vi "Single Engine Main.vi"() -> ()   [LabVIEW 2013]
uses:
  <vilib>/NI/Module Execution Interface/Engine Runtime/Execution States.ctl
  <vilib>/NI/Module Execution Interface/Engine Runtime/Engine Runtime Interface.lvclass
  Framework Configuration Classes/target runtime/PL_Target Runtime.lvclass
  Framework Configuration Classes/platypus configuration/PLConfigurationSerializer.lvlib
  <vilib>/rvi/interface/nirviOpenFPGA/nirviOpenFPGA.xnode
  <vilib>/NI/Tag Bus Module Framework/FPGA manager/FPGA manager.lvlib
  <vilib>/NI/Tag Bus Module Framework/FPGA manager/methods.ctl
  <vilib>/userdefined/High Color/nirio_resource_hc.ctl
panel:
  out "final error":errorcluster
  in  "stop":bool
  out "runtime error":errorcluster
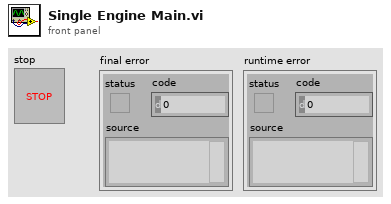
[diagram p1: front panel]
types:
  T1 = typedef "nirio_resource_hc.ctl" = tag
  T2 = typedef "FPGA manager.lvlib/methods.ctl" = enum16{"initialize bitfile", "cache bitfile", "locate bitfile", "close bitfile"}
  T3 = typedef "PLConfigurationSerializer.lvlib/file format.ctl" = cluster{"version":string, "data":string}
  T4 = typedef "PLConfigurationSerializer.lvlib/1_0_0_0 format.ctl" = cluster{"system":T5, "database":T8[]}
  T5 = typedef "PLConfigurationSerializer.lvlib/system hierarchy.ctl" = cluster{"system ID":string, "targets":T6[]}
  T6 = typedef "PLConfigurationSerializer.lvlib/target hierarchy.ctl" = cluster{"target ID":string, "engines":T7[]}
  T7 = typedef "PLConfigurationSerializer.lvlib/engine hierarchy.ctl" = cluster{"engine ID":string, "modules IDs":string[]}
  T8 = typedef "PLConfigurationSerializer.lvlib/configuration database.ctl" = cluster{"ID":string, "display name":string, "class":string, "version":string, "data":string}
  T9 = typedef "PLConfigurationSerializer.lvlib/targets cluster.ctl" = cluster{"Target Configuration":refnum<class "PL_Target Configuration.lvclass">, "engines":T10[]}
  T10 = typedef "PLConfigurationSerializer.lvlib/engines cluster.ctl" = cluster{"engine configuration":refnum<class "engine configuration.lvclass">, "modules":refnum<class "TBM module configuration.lvclass">[]}
  T11 = typedef "Engine Runtime Interface.lvclass/Execution States.ctl" = enum16{"Initializing", "Paused (Initialized)", "Running", "Set Safe Outputs", "Uninitializing", "Stopped (Uninitialized)", "Error (Uninitialized)", "Safe State (Uninitialized)", "Closed"}
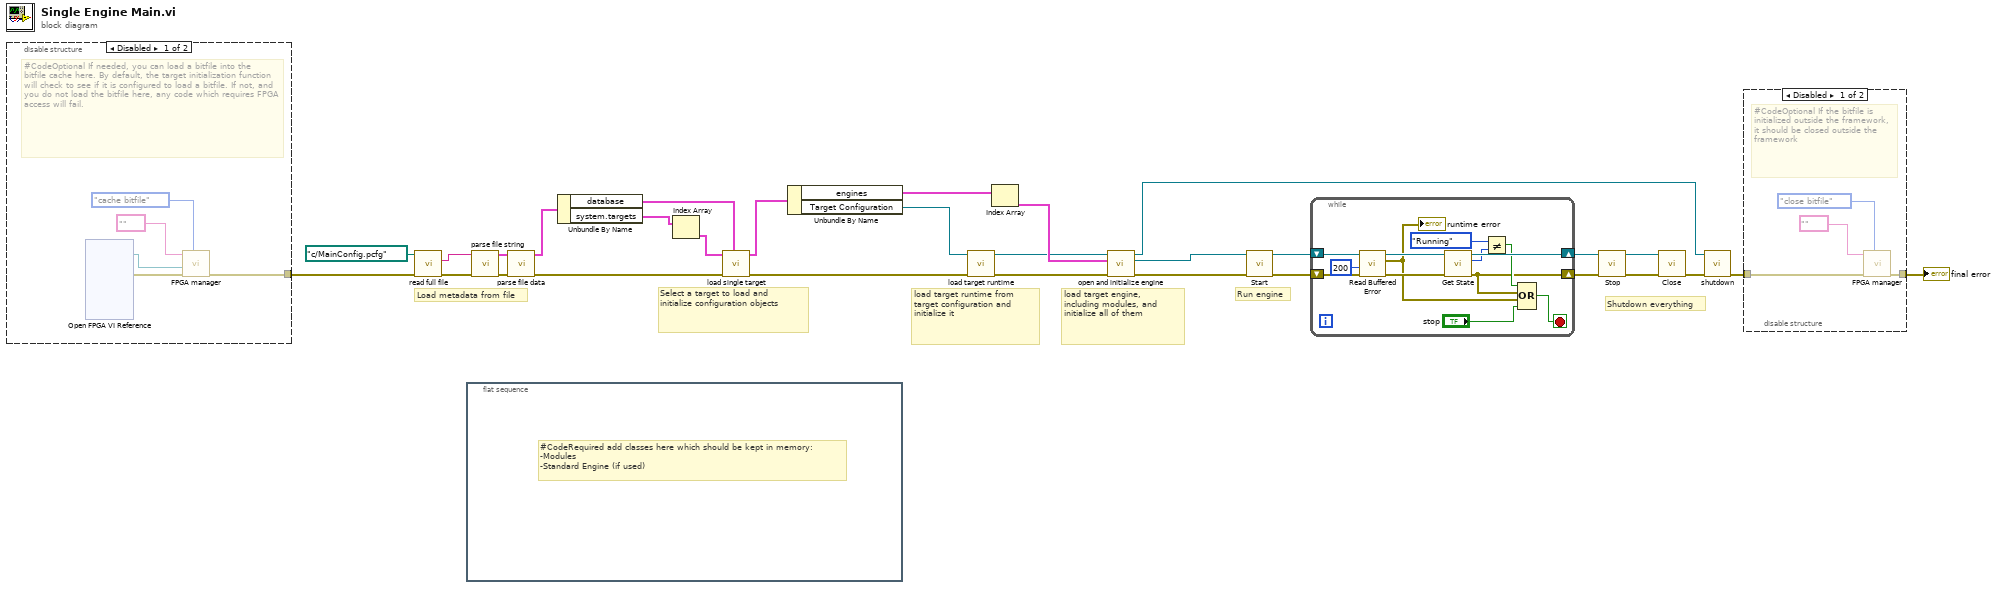
[diagram p0: block diagram]
diagram:
  # "Shutdown everything"
  # "Run engine"
  # "load target engine, including modules, and initialize all of them"
  # "load target runtime from target configuration and initialize it"
  # "Select a target to load and initialize configuration objects"
  # "Load metadata from file"
  n1 = disable-structure shown="Disabled" {
    disable-tunnel: [w31 _] -> w3
    frame Disabled {
      # "#CodeOptional If needed, you can load a bitfile into the bitfile cache here. By default, the target initialization function will check to see if it is configured to load a bitfile. If not, and you do not load the bitfile here, any code which requires FPGA access will fail."
      n2 = xnode "Open FPGA VI Reference"() -> ("FPGA VI Reference Out"=w34:refnum<k20>, "error out"=w35:errorcluster)  [unwired: 2 in]
      n3 = call <vilib>:"FPGA manager.vi"("action"=methods."cache bitfile", "error in"=w35, "bitfile to cache"=w34, "RIO resource"=T1 "") -> ("error out"=w31:errorcluster)  [unwired: 5 in, 2 out]
    }
    frame Enabled {
    }
  }
  n4 = call "read full file.vi"("error in"=w3, "file path"=path "c:/MainConfig.pcfg") -> ("error out"=w20:errorcluster, "data"=w21:string)  [unwired: 8 in]
  n5 = flat-sequence {
    frame #0 {
      # "#CodeRequired add classes here which should be kept in memory:\n-Modules\n-Standard Engine (if used)"
      # "Add classes here to be in memory"
    }
  }
  n6 = call "parse file string.vi"("error in"=w20, "data string"=w21) -> ("error out"=w22:errorcluster, "file format"=w23:T3)  [unwired: 8 in]
  n7 = call "parse file data.vi"("error in"=w22, "file format"=w23) -> ("error out"=w18:errorcluster, "file information"=w19:T4)  [unwired: 8 in]
  n8 = Unbundle By Name(w19) -> ("database"=w17:T8[], "system.targets"=w16:T6[])
  n9 = Index Array(array=w16) -> (element=w15:T6)  [unwired: 1 in]
  n10 = call "load single target.vi"("database in"=w17, "error in"=w18, "target to load"=w15) -> ("error out"=w6:errorcluster, "targets cluster out"=w14:T9)  [unwired: 7 in]
  n11 = Unbundle By Name(w14) -> ("engines"=w13:T10[], "Target Configuration"=w7:refnum<class "PL_Target Configuration.lvclass">)
  n12 = call "load target runtime.vi"("error in"=w6, "target configuration"=w7) -> ("error out"=w5:errorcluster, "target runtime"=w4:refnum<class "PL_Target Runtime.lvclass">)  [unwired: 8 in]
  n13 = Index Array(array=w13) -> (element=w8:T10)  [unwired: 1 in]
  n14 = call "open and initialize engine.vi"("error in"=w5, "engine configuration in"=w8, "Target Runtime in"=w4) -> ("error out"=w12:errorcluster, "Engine Runtime Interface out"=w11:refnum<class "Engine Runtime Interface.lvclass">, "Target Runtime out"=w9:refnum<class "PL_Target Runtime.lvclass">)  [unwired: 6 in]
  n15 = call-dynamic "Start.vi"("error in"=w12, "Engine Runtime Interface in"=w11) -> ("error out"=w24:errorcluster, "Engine Runtime Interface out"=w27:refnum<class "Engine Runtime Interface.lvclass">)  [unwired: 8 in]
  n16 = while {
    shift-right: [w44] -> w26
    shift-left: w27 -> [w48]
    shift-right: [w37] -> w25
    shift-left: w24 -> [w47]
    stop <- w42 stop-if-true
    n17 = call-dynamic "Read Buffered Error.vi"("error in"=w47, "timeout in ms (0)"=200, "Engine Runtime Interface in"=w48) -> ("error out"=w45:errorcluster, "Engine Error"=w41:errorcluster, "Engine Runtime Interface out"=w46:refnum<class "Engine Runtime Interface.lvclass">)  [unwired: 6 in]
    "runtime error" <- w41
    n18 = call-dynamic "Get State.vi"("error in"=w45, "Engine Runtime Interface in"=w46) -> ("error out"=w37:errorcluster, "Engine State"=w40:T11, "Engine Runtime Interface out"=w44:refnum<class "Engine Runtime Interface.lvclass">)  [unwired: 7 in]
    n19 = Not Equal?(x=Execution_States."Running" ("Engine State"), y=w40) -> (x != y?=w38:bool)
    n20 = Compound Arithmetic op=OR(w38, w37, w41, "stop") -> (w42:bool)
  }
  n21 = call-dynamic "Stop.vi"("error in"=w25, "Engine Runtime Interface in"=w26) -> ("error out"=w28:errorcluster, "Engine Runtime Interface out"=w29:refnum<class "Engine Runtime Interface.lvclass">)  [unwired: 8 in]
  n22 = call-dynamic "Close.vi"("error in"=w28, "Engine Runtime Interface in"=w29) -> ("error out"=w10:errorcluster)  [unwired: 9 in]
  n23 = call-dynamic "shutdown.vi"("error in"=w10, "Target Runtime in"=w9) -> ("error out"=w2:errorcluster)  [unwired: 9 in]
  n24 = disable-structure shown="Disabled" {
    disable-tunnel: w2 -> [w50 w53]
    disable-tunnel: [w49 w53] -> w1
    frame Disabled {
      # "#CodeOptional If the bitfile is initialized outside the framework, it should be closed outside the framework"
      n25 = call <vilib>:"FPGA manager.vi"("action"=methods."close bitfile", "error in"=w50, "RIO resource"=T1 "") -> ("error out"=w49:errorcluster)  [unwired: 6 in, 2 out]
    }
    frame Enabled {
    }
  }
  "final error" <- w1
